vi "Reject invalid cam video data.vi"(9 "Acquisition time unknown":bool, 10 "Experiment Header's Statistics":T1, 11 "Cam video's timestamps file":i64[][](array[numeric])) -> (1 "Frame relative times array":i64[](array[numeric]), 2 "Number of original frames":i32, 3 "Frame numbers array":i64[](array[numeric]), 4 "Elements to keep":bool[](array[boolean]))   [LabVIEW 2020]
uses:
  Typedefs/Test header stats cluster.ctl
  <userlib>/_OpenG.lib/array/array.llb/Conditional Auto-Indexing Tunnel (I64)__ogtk.vi
panel:
  out "Number of valid frames":i32
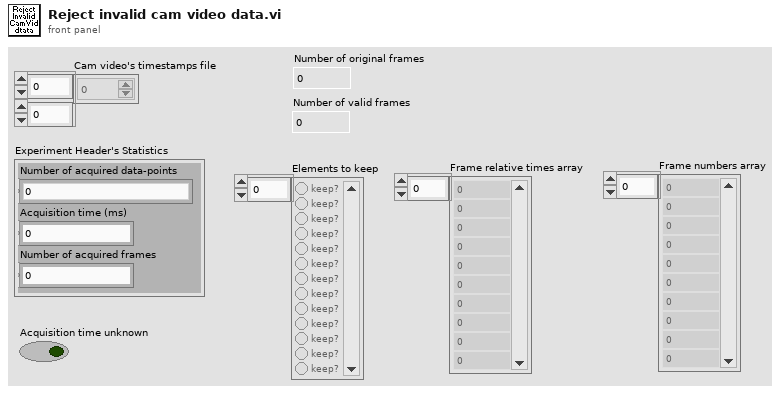
[diagram p1: front panel]
types:
  T1 = typedef "Test header stats cluster.ctl" = cluster{"Number of acquired data-points":dbl, "Acquisition time (ms)":dbl, "Number of acquired frames":dbl}
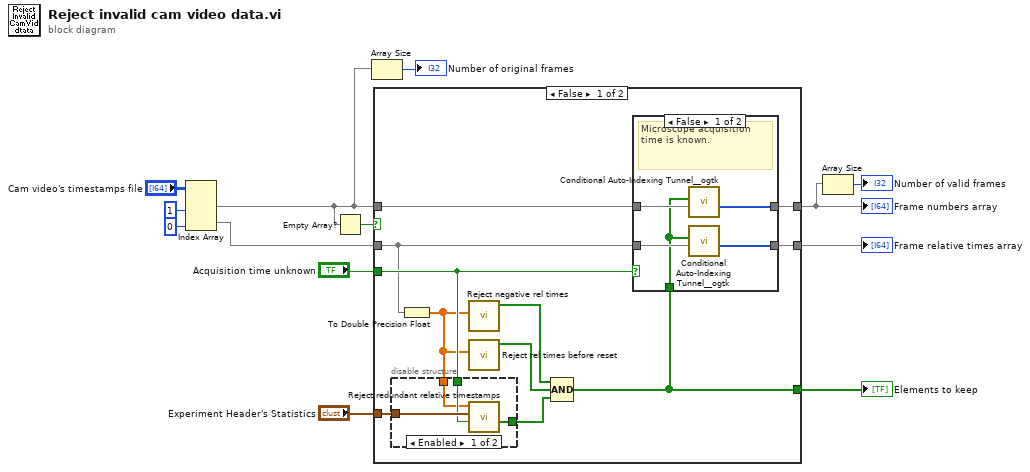
[diagram p0: block diagram]
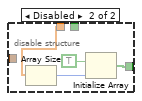
[diagram p2: hidden frame]
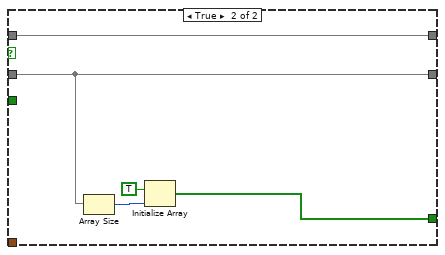
[diagram p4: hidden frame]
diagram:
  n1 = Index Array(array="Cam video's timestamps file", index (col) #1=1 ("disabled index (col)"), index (col) #2=0 ("index (row)")) -> (element #1=w3:i64[], element #2=w7:i64[])  [unwired: 2 in]
  n2 = Empty Array?(array=w3) -> (empty?=w10:bool)
  n3 = Array Size(array=w3) -> (size(s)=→"Number of original frames":i32)
  n4 = case shown="False" w10 {
    tunnel: w3 -> [w24 w44]
    tunnel: [w23 w44] -> w1
    tunnel: w7 -> [w16 w40]
    tunnel: "Experiment Header's Statistics" -> [w22 _]
    tunnel: "Acquisition time unknown" -> [w18 _]
    tunnel: [w20 w41] -> w9
    tunnel: [w19 w40] -> w8
    frame False {
      n5 = To Double Precision Float(number=w16) -> (double precision float=w15:dbl[])
      n6 = disable-structure shown="Enabled" {
        disable-tunnel: w22 -> [w28 _]
        disable-tunnel: [w27 w29] -> w21
        disable-tunnel: w18 -> [w26 _]
        disable-tunnel: w15 -> [w25 w30]
        frame Enabled {
          n7 = call "Reject redundant relative timestamps.vi"("Acquisition time unknown"=w26, "Experiment Header's Statistics"=w28, "Frame relative times array"=w25) -> ("Elements to keep"=w27:bool[])  [unwired: 5 in, 3 out]
        }
        frame Disabled {
          n8 = Array Size(array=w30) -> (size(s)=w31:i32)
          n9 = Initialize Array(TRUE ("No test header file"), w31) -> (w29:bool[])
        }
      }
      n10 = call "Reject negative rel times.vi"("Timestamps (ms)"=w15) -> ("Keep"=w14:bool[])  [unwired: 10 in]
      n11 = call "Reject rel times before reset.vi"("Timestamps (ms)"=w15) -> ("Keep"=w17:bool[])  [unwired: 10 in]
      n12 = Compound Arithmetic op=AND(w14, w17, w21) -> (w20:bool[])
      n13 = case shown="False" w18 {
        tunnel: w24 -> [w37 w39]
        tunnel: [w36 w39] -> w23
        tunnel: w20 -> [w33 _]
        tunnel: w16 -> [w35 w38]
        tunnel: [w34 w38] -> w19
        frame False {
          # "Microscope acquisition time is known."
          n14 = call-poly <userlib>:"Conditional Auto-Indexing Tunnel__ogtk.vi"("Array in"=w37, "Elements to keep"=w33) -> ("Filtered Array out"=w36:i64[])  [unwired: 5 in]
          n15 = call-poly <userlib>:"Conditional Auto-Indexing Tunnel__ogtk.vi"("Array in"=w35, "Elements to keep"=w33) -> ("Filtered Array out"=w34:i64[])  [unwired: 5 in]
        }
        frame True {
          # "Microscope acquisition time unknown."
        }
      }
    }
    frame True {
      n16 = Array Size(array=w40) -> (size(s)=w42:i32)
      n17 = Initialize Array(TRUE ("No test header file"), w42) -> (w41:bool[])
    }
  }
  "Frame relative times array" <- w8
  "Frame numbers array" <- w1
  "Elements to keep" <- w9
  n18 = Array Size(array=w1) -> (size(s)=→"Number of valid frames":i32)
